vi "Check Should Log.vi"(6 "LogLevel":T1, 11 "Log Sink in":refnum<class "Log Sink.lvclass">) -> (3 "Log Sink out":refnum<class "Log Sink.lvclass">, 4 "Log?":bool)   [LabVIEW 2019, in "Composed Log.lvlib" / "Log Sink.lvclass"]
uses:
  <vilib>/gpm_packages/@cs/event-logger/Source/Composed Log/Log Sink/Log Sink.lvclass
  <vilib>/gpm_packages/@cs/event-logger/Source/Composed Log/Types/Log Level.ctl
  <vilib>/gpm_packages/@cs/event-logger/Source/Composed Log/Log Sink/Log Sink.lvclass/Log Sink.ctl
  <vilib>/gpm_packages/@cs/event-logger/Source/Composed Log/Composed Log.lvlib
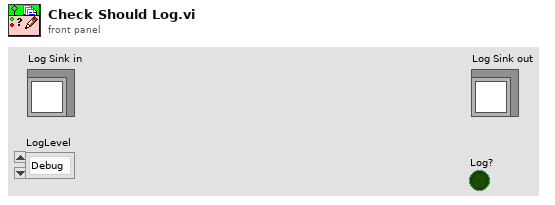
[diagram p1: front panel]
types:
  T1 = typedef "Composed Log.lvlib/Log Level.ctl" = enum16{"Debug", "Info", "Warning", "Error", "Critical"}
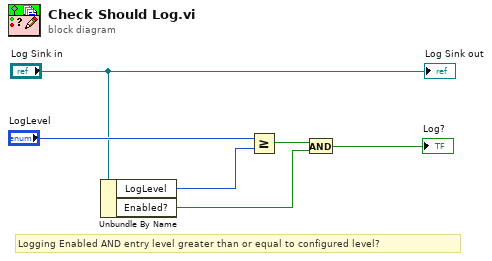
[diagram p0: block diagram]
diagram:
  # "Logging Enabled AND entry level greater than or equal to configured level?"
  n1 = Unbundle By Name("Log Sink in") -> ("LogLevel"=w5:T1, "Enabled?"=w3:bool)
  n2 = Greater Or Equal?(x="LogLevel", y=w5) -> (x >= y?=w4:bool)
  n3 = And(x=w4, y=w3) -> (x .and. y?=→"Log?":bool)
  "Log Sink out" <- "Log Sink in"
